vi "Ensure Cursor in ROI.vi"(8 "error in":errorcluster, 11 "Base Graph in":refnum<class "Base Graph.lvclass">) -> (0 "error out":errorcluster, 3 "Base Graph out":refnum<class "Base Graph.lvclass">)   [LabVIEW 2023, in "Base Graph.lvclass"]
uses:
  Base Graph.lvclass
  Base Graph.lvclass/Base Graph.ctl
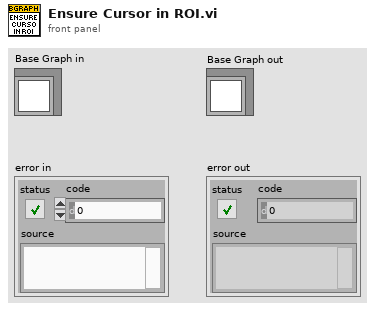
[diagram p1: front panel]
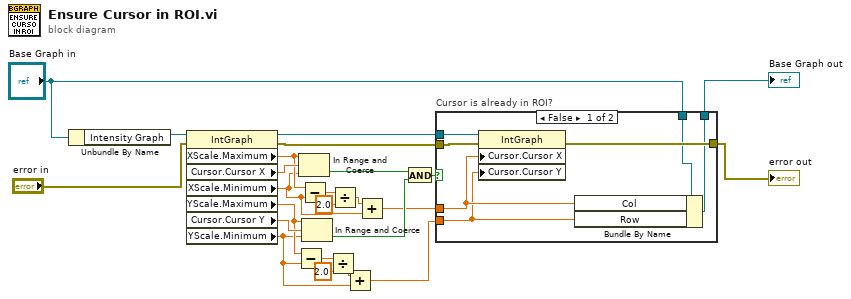
[diagram p0: block diagram]
diagram:
  n1 = Unbundle By Name("Base Graph in") -> ("Intensity Graph"=w24:refnum<vi>)
  n2 = property class="IntGraph"(reference=w24, error in="error in") -> (reference out=w20:refnum<vi>, error out=w3:errorcluster, "XScale.Maximum"=w22:dbl, "Cursor.Cursor X"=w23:dbl, "XScale.Minimum"=w11:dbl, "YScale.Maximum"=w17:dbl, "Cursor.Cursor Y"=w18:dbl, "YScale.Minimum"=w14:dbl)
  n3 = Subtract(x=w17, y=w14) -> (x-y=w16:dbl)
  n4 = In Range and Coerce(upper limit=w22, x=w23, lower limit=w11) -> (In Range?=w8:bool)  [unwired: 1 out]
  n5 = Subtract(x=w22, y=w11) -> (x-y=w19:dbl)
  n6 = In Range and Coerce(upper limit=w17, x=w18, lower limit=w14) -> (In Range?=w9:bool)  [unwired: 1 out]
  n7 = Divide(x=w16, y=2.0) -> (x/y=w13:dbl)
  n8 = Divide(x=w19, y=2.0) -> (x/y=w12:dbl)
  n9 = Add(x=w13, y=w14) -> (x+y=w6:dbl)
  n10 = Add(x=w12, y=w11) -> (x+y=w7:dbl)
  n11 = And(x=w8, y=w9) -> (x .and. y?=w10:bool)
  n12 = case "Cursor is already in ROI?" shown="False" w10 {
    tunnel: w20 -> [w31 _]
    tunnel: w7 -> [w26 _]
    tunnel: w6 -> [w25 _]
    tunnel: [w30 w33] -> w5
    tunnel: w3 -> [w29 w33]
    tunnel: "Base Graph in" -> [w28 w32]
    tunnel: [w27 w32] -> w1
    frame False {
      n13 = property class="IntGraph"(reference=w31, error in=w29, "Cursor.Cursor X"=w26, "Cursor.Cursor Y"=w25) -> (error out=w30:errorcluster)  [unwired: 1 out]
      n14 = Bundle By Name(cluster=w28, "Col"=w26, "Row"=w25) -> (w27:refnum<class "Base Graph.lvclass">)
    }
    frame True {
    }
  }
  "error out" <- w5
  "Base Graph out" <- w1
